vi "test_fpga.vi"() -> ()   [LabVIEW 2013]
uses:
  <vilib>/rvi/DesktopExecutionNode/Execution/niFpgaDEN_Execute.vi
  <vilib>/rvi/DesktopExecutionNode/DesktopExecutionNode.xnode
panel:
  out "ch0 2":dbl(graph)
  out "ch2 2":dbl(graph)
  out "ch1 2":dbl(graph)
  in  "stop":bool
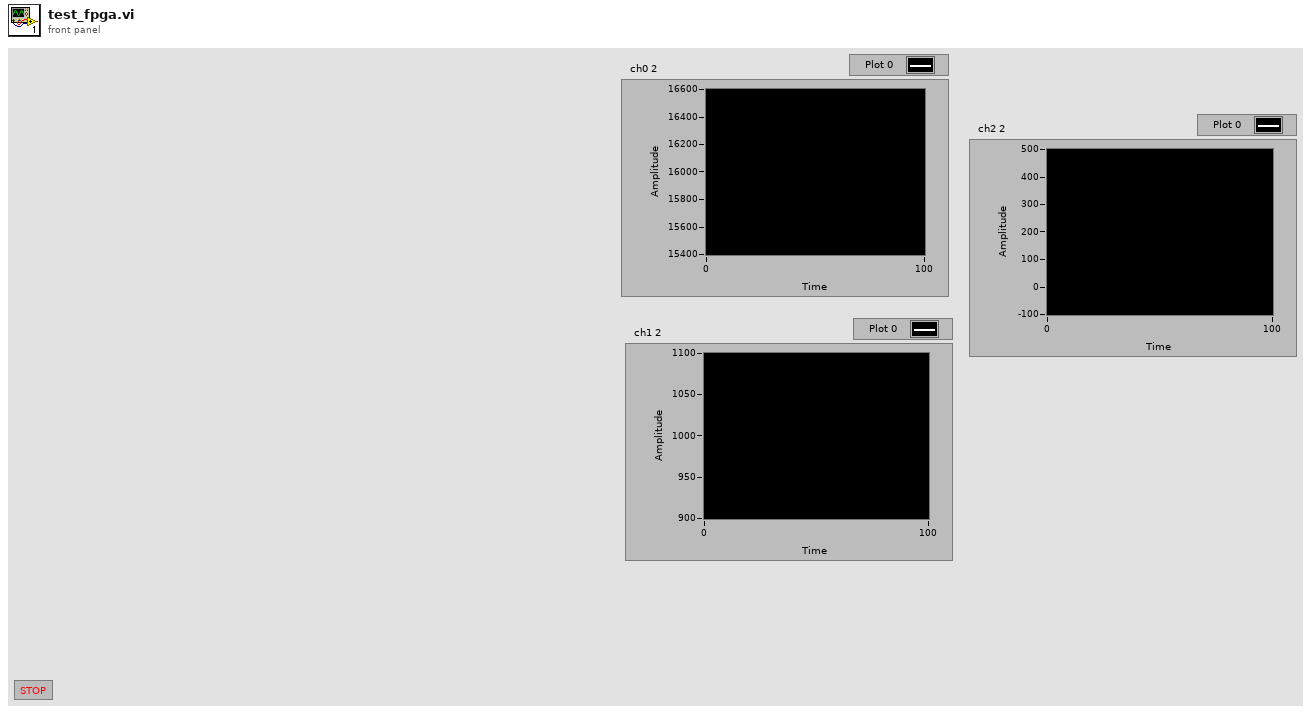
[diagram p1: front panel]
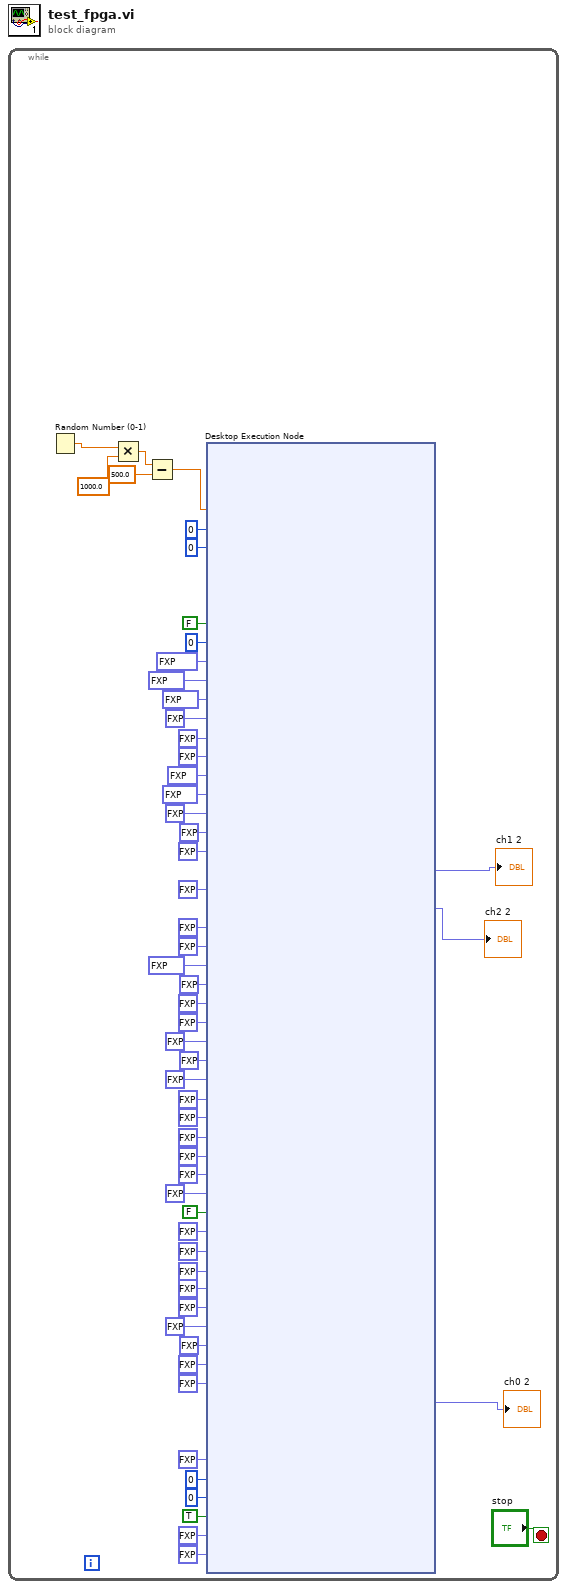
[diagram p0: block diagram]
diagram:
  n1 = while {
    stop <- "stop" stop-if-true
    n2 = Random Number (0-1)() -> (number: 0 to 1=w7:dbl)
    n3 = Multiply(x=w7, y=1000.0) -> (x*y=w5:dbl)
    n4 = Subtract(x=w5, y=500.0) -> (x-y=w3:dbl)
    n5 = xnode "Desktop Execution Node"("AI0"=w3, "Connector0/AI2"=i16 0, "Connector0/AI1"=i16 0, "Stop"=FALSE, "Count(uSec)"=u32 0, "Lower lim 0"=fxp<+/-,32,16> -10000.0, "Upper lim 0"=fxp<+/-,32,16> 10000.0, "Dc offset 0"=fxp<+/-,32,16> 15500.0, "pg 0"=fxp<+/-,32,16> 1.0, "dg 0"=fxp<+/-,32,16> 0.0, "Setpoint 1"=fxp<+/-,16,16> 0.0, "Lower lim 1"=fxp<+/-,32,16> 1000.0, "Upper lim 1"=fxp<+/-,32,16> -1000.0, "Dc offset 1"=fxp<+/-,32,16> 0.0, "pg 1"=fxp<+/-,32,16> 0.0, "dg 1"=fxp<+/-,32,16> 0.0, "Dc Pos 2"=fxp<+/-,32,16> 0.0, "pg 2"=fxp<+/-,32,16> 1.0, "dg 2"=fxp<+/-,32,16> 0.0, "Upper lim 2"=fxp<+/-,32,16> 32000.0, "Lower lim 2"=fxp<+/-,32,16> 0.0, "Dc offset 2"=fxp<+/-,32,16> 0.0, "1,1"=fxp<+/-,32,16> 1.0, "1, 2"=fxp<+/-,32,16> 0.0, "1, 3"=fxp<+/-,32,16> 0.0, "2, 1"=fxp<+/-,32,16> 0.0, "2, 2"=fxp<+/-,32,16> 1.0, "2, 3"=fxp<+/-,32,16> 0.0, "3, 3"=fxp<+/-,32,16> 1.0, "3, 2"=fxp<+/-,32,16> 0.0, "3, 1"=fxp<+/-,32,16> 0.0, "frequency (periods/tick)"=fxp<+,32,0> 0.0, "reset freq"=FALSE, "Drive_gain 0"=fxp<+/-,32,16> 0.0, "Zfb norm const 0"=fxp<+/-,32,16> 1.0, "Z offset 0"=fxp<+/-,32,16> 1.0, "Dc Pos 0"=fxp<+/-,32,16> 0.0, "meters per bit beam displacement 0"=fxp<+/-,32,16> 1.0, "Dc Pos 1"=fxp<+/-,32,16> 1.0, "Drive_gain 1"=fxp<+/-,32,16> 0.0, "Z offset 1"=fxp<+/-,32,16> 1.0, "meters per bit beam displacement 1"=fxp<+/-,32,16> 1.0, "Zfb norm const"=fxp<+/-,32,16> 0.0, "RMS 1 (bits)"=u16 0, "RMS 0 (bits)"=u16 0, "apply corrections"=TRUE, "meters per measured bit 1"=fxp<+/-,32,16> 1.0, "meters per measured bit 0"=fxp<+/-,32,16> 1.0) -> ("fb+dc+drive_1"=→"ch1 2":fxp<+/-,32,16>, "fb +dc_2"=→"ch2 2":fxp<+/-,32,16>, "fb+dc+drive_0"=→"ch0 2":fxp<+/-,48,32>)  [unwired: 1 in, 6 out]
  }
